vi "FPGA_Lock-In (1).vi"() -> ()   [LabVIEW 2012]
panel:
  in  "Numeric 2":dbl
  out "Partial Phase":dbl
  out "Phase Shift Difference":dbl
  out "P1":dbl
  out "P2":dbl
  out "Numeric":dbl
  out "Waveform Chart 2":dynamicdata(graph)
  out "Waveform Chart":dynamicdata(graph)
  in  "stop":bool
  out "Freq":dbl
  out "Amp_Signal":dbl
  out "Freq":dbl
  out "Amp_Ref":dbl
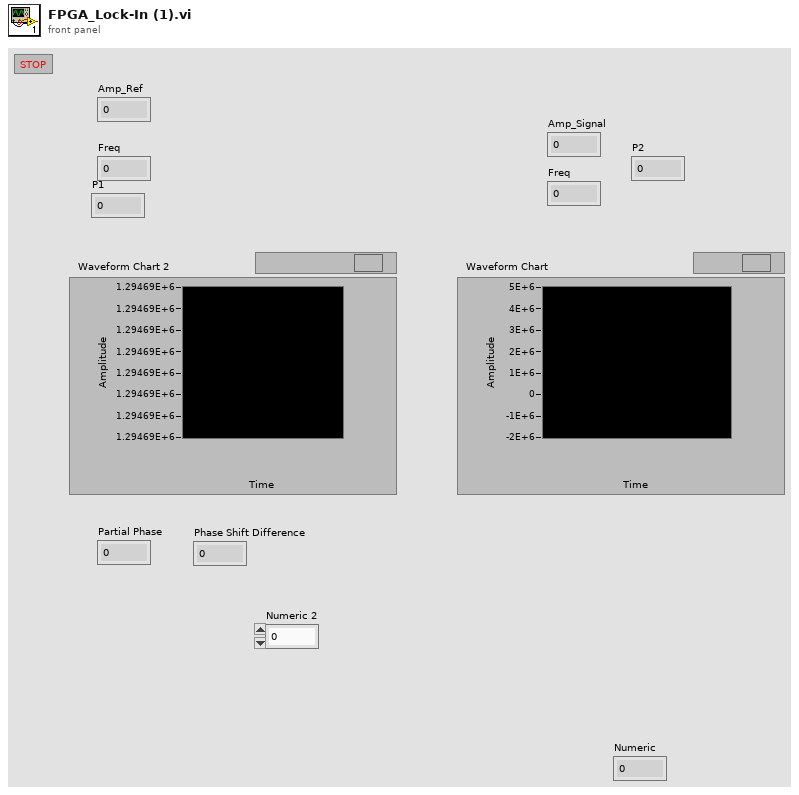
[diagram p1: front panel]
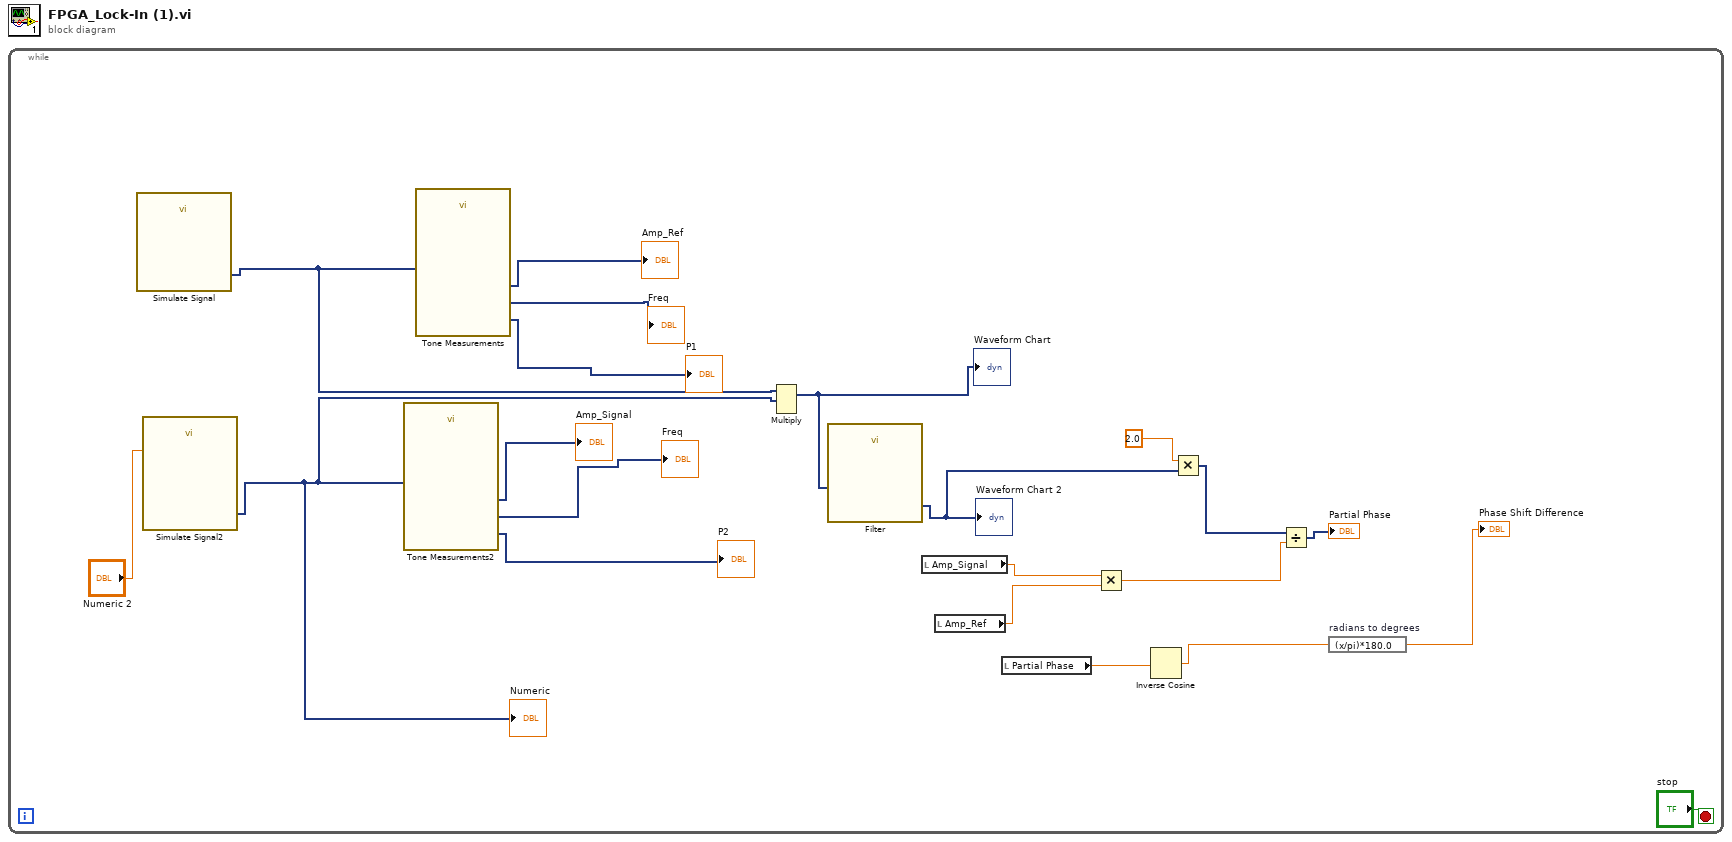
[diagram p0: block diagram]
diagram:
  n1 = while {
    stop <- "stop" stop-if-true
    n2 = call "Simulate Signal"() -> ("Sine"=w16:dynamicdata)  [unwired: 14 in, 1 out]
    n3 = call "Simulate Signal2"("Phase"="Numeric 2") -> ("Sine"=w14:dynamicdata)  [unwired: 13 in, 1 out]
    "Numeric" <- w14
    n4 = call "Tone Measurements2"("Signals"=w14) -> ("Phase"=→"P2":dynamicdata, "Frequency"=→"Freq":dynamicdata, "Amplitude"=→"Amp_Signal":dynamicdata)  [unwired: 7 in, 1 out]
    n5 = call "Tone Measurements"("Signals"=w16) -> ("Phase"=→"P1":dynamicdata, "Frequency"=→"Freq":dynamicdata, "Amplitude"=→"Amp_Ref":dynamicdata)  [unwired: 7 in, 1 out]
    n6 = Multiply(1:w14, 2:w16) -> (0:w15:dynamicdata)  [unwired: 1 in, 1 out]
    "Waveform Chart" <- w15
    n7 = call "Filter"("Signal"=w15) -> ("Filtered Signal"=w10:dynamicdata)  [unwired: 9 in, 1 out]
    "Waveform Chart 2" <- w10
    n8 = local read "Amp_Signal"() -> (w9:dbl)
    n9 = local read "Amp_Ref"() -> (w8:dbl)
    n10 = local read "Partial Phase"() -> (w4:dbl)
    n11 = Multiply(x=w9, y=w8) -> (x*y=w6:dbl)
    n12 = Inverse Cosine(1:w4) -> (0:w3:dbl)
    n13 = Multiply(x=2.0, y=w10) -> (x*y=w7:dynamicdata)
    n14 = Divide(x=w7, y=w6) -> (x/y=→"Partial Phase":dynamicdata)
    n15 = expression code="(x/pi)*180.0" "radians to degrees"(w3) -> (→"Phase Shift Difference":dbl)
  }
